vi "5668 Stop Scan with External LO.vi"(8 "error in (no error)":errorcluster, 10 "RFSG Instrument Handle In":refnum<k15>, 11 "RFSA Instrument Handle In":refnum<k15>) -> (0 "error out":errorcluster)   [LabVIEW 2017]
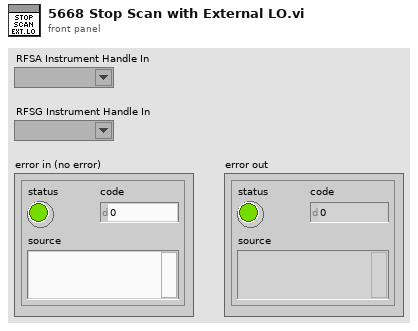
[diagram p1: front panel]
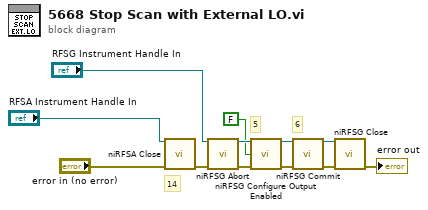
[diagram p0: block diagram]
diagram:
  # "6"
  # "5"
  # "14"
  n1 = call <instrlib>:"niRFSA Close.vi"("instrument handle"="RFSA Instrument Handle In", "error in"="error in (no error)") -> ("error out"=w10:errorcluster)  [unwired: 13 in]
  n2 = call <instrlib>:"niRFSG Abort.vi"("instrument handle"="RFSG Instrument Handle In", "error in"=w10) -> ("instrument handle out"=w8:refnum<k15>, "error out"=w9:errorcluster)  [unwired: 12 out]
  n3 = call <instrlib>:"niRFSG Configure Output Enabled.vi"("instrument handle"=w8, "output enabled"=FALSE ("output enable"), "error in"=w9) -> ("instrument handle out"=w4:refnum<k15>, "error out"=w5:errorcluster)  [unwired: 11 out]
  n4 = call <instrlib>:"niRFSG Commit.vi"("instrument handle"=w4, "error in"=w5) -> ("instrument handle out"=w7:refnum<k15>, "error out"=w6:errorcluster)  [unwired: 12 out]
  n5 = call <instrlib>:"niRFSG Close.vi"("instrument handle"=w7, "error in"=w6) -> ("error out"=→"error out":errorcluster)  [unwired: 13 out]
